vi "_sp_spurious.vi"(11 "SP_Spurious":cluster{"Rx_output_data":path, "SAVE":bool}={"Rx_output_data"=path "L:/cartridge/assembly/SN03/03-23/111227_DSB/SP_810.00_120_111227_CCA03-23_DSBFB.csv", "SAVE"=TRUE}) -> (1 "出力文字列":string="SP_spurious,0.82,4.01,-33.89,-32.15 ")   [LabVIEW 2017]
uses:
  <vilib>/Utility/file.llb/Read From Spreadsheet File (string).vi
panel:
  out "配列 2":dbl[][](array[numeric])=[[3.8, -17.12272, -18.81083, -15.55195, -27.42913, -0.8529618823529413, 2646.4699989426, 27.159200000349998, 21.830696906606043], [3.85, -17.57263, -19.57423, -15.61331, -27.39271, -0.8547822352941177, 2630.0700003280003, 27.222799998728, 21.827656711269793], [3.9, -17.18393, -19.46044, -15.25915, -26.95194, -0.8662073529411765, 2669.6499992084, 27.104500002366002, 21.82485128829734], [3.95, -16.20817, -18.50417, -14.57025, -26.2268, -0.8667218823529415, 2730.9599987738, 27.08000000049, 21.822294447827726], [4.0, -15.03429, -17.26599, -13.90883, -25.64848, -0.882467, 2669.1500012362003, 27.084199999916, 21.82], [4.05, -14.82404, -17.0148, -13.89065, -25.63071, -0.881857, 2537.9100026248, 27.120499999274, 21.817975444814163], [4.1, -14.67198, -16.88321, -13.75199, -25.74328, -0.8925589411764706, 2521.6700003248, 26.984300002724, 21.81620304171403], [4.15, -13.82526, -16.05723, -13.35155, -25.22083, -0.8985360624999998, 2529.2999998474, 26.948000000726, 21.81465874000436], [4.2, -13.29308, -15.43659, -13.22012, -25.15282, -0.901060705882353, 2508.1700004226, 26.933300000294, 21.81331848898993], [4.25, -13.22027, -15.33436, -13.24037, -25.05297, -0.9175218823529412, 2527.4499996144, 26.893400000798, 21.812158237975495], [4.3, -13.31871, -15.44813, -13.02047, -24.85233, -0.9171115294117648, 2617.4499981999998, 26.800200001864, 21.81115393626583], [4.35, -13.69981, -15.96198, -12.64103, -24.38364, -0.9331128235294116, 2655.3199992426003, 26.946899997065998, 21.810281533165693], [4.4, -13.88617, -16.39624, -12.56773, -24.29817, -0.9225989999999998, 2612.6100008542003, 26.89840000097, 21.809516977979857], [4.45, -14.02675, -16.71935, -12.80309, -24.58885, -0.9326420000000001, 2578.7800006766, 26.85540000086, 21.808836220013085], [4.5, -14.20917, -16.89711, -12.97901, -24.88372, -0.9390088823529412, 2494.6900016818004, 26.752700002054002, 21.808215208570147], [4.55, -14.08214, -16.69081, -12.94844, -24.93315, -0.948472375, 2435.9600011746, 26.64920000207, 21.807629892955802], [4.6, -14.17748, -16.75517, -13.06879, -25.00575, -0.9494775294117647, 2433.2400000544, 26.427400004436, 21.80705622247482], [4.65, -14.20809, -16.81901, -13.13087, -25.16717, -0.9524575882352941, 2443.0399998039998, 26.363500001278, 21.80647014643197], [4.7, -13.73884, -16.38887, -13.13099, -25.03512, -0.9655740588235294, 2433.8500001838, 26.45199999823, 21.805847614132016], [4.75, -13.52419, -16.15298, -13.15192, -24.9704, -0.9653059411764703, 2516.0199983566, 26.454299999954, 21.805164574879722], [4.8, -13.5663, -16.20232, -13.10517, -24.80095, -0.976770176470588, 2562.8099990642, 26.343600002214, 21.804396977979856], [4.85, -13.97629, -16.65383, -13.30715, -25.25404, -0.9746549411764707, 2478.4000016882, 26.311400000644, 21.803520772737187], [4.9, -14.61364, -17.38417, -13.78671, -25.66877, -0.988881117647059, 2394.9800016684003, 26.140100003426, 21.802511908456477], [4.95, -14.4268, -17.25931, -13.81209, -25.80221, -0.9904888125, 2426.7199993652, 26.145399999894, 21.801346334442492], [5.0, -13.84685, -16.67325, -13.20797, -25.09457, -0.9986477647058825, 2402.3700004869997, 26.405599994796, 21.8], [5.05, -14.28601, -17.05717, -13.45101, -25.54052, -1.004, 2304.7500019524, 26.325300001606, 21.798457844989954], [5.1, -14.91876, -17.64101, -13.96415, -26.02207, -1.0068823529411761, 2324.9199995966, 26.481899996868, 21.796740771498058], [5.15, -15.14906, -17.85047, -14.16308, -26.17572, -1.0180588235294117, 2408.1599983352, 26.271100004216002, 21.794878672166195], [5.2, -14.66069, -17.39484, -13.82115, -25.80543, -1.0208823529411764, 2393.2200002987997, 26.329699998827998, 21.792901439636257], [5.25, -13.73691, -16.45963, -13.31747, -25.36704, -1.028, 2326.370001337, 26.25120000157, 21.790838966550133], [5.3, -13.70664, -16.41934, -13.34713, -25.41262, -1.0291176470588232, 2366.9299991887997, 26.28519999932, 21.78872114554971], [5.35, -14.26567, -16.97919, -13.7311, -25.69348, -1.042, 2383.6799996649997, 26.357999998544, 21.78657786927688], [5.4, -14.42577, -17.17993, -13.89956, -26.00954, -1.046, 2311.580001442, 26.332800000503997, 21.784439030373523], [5.45, -14.3035, -17.10186, -13.87839, -26.01249, -1.0538235294117648, 2274.08000075, 26.241800001820003, 21.782334521481534], [5.5, -14.13436, -16.92141, -13.94402, -26.09274, -1.0542500000000001, 2305.5199993712, 26.224000000356, 21.780294235242803], [5.55, -14.09064, -16.88934, -13.93655, -25.97309, -1.0640588235294117, 2314.2099998262, 26.143600001608, 21.778348064299216], [5.6, -14.13487, -16.88146, -13.83602, -26.02727, -1.0725882352941176, 2258.5000011142, 26.194499998982, 21.776525901292658], [5.65, -14.0179, -16.75543, -13.67357, -25.85477, -1.0641764705882353, 2249.6300001774002, 26.303699997816, 21.774857638865026], [5.7, -13.742, -16.4761, -13.49645, -25.65245, -1.085294117647059, 2312.4099987443997, 26.495899996156, 21.7733731696582], [5.75, -13.63401, -16.37811, -13.62051, -25.66763, -1.0879411764705882, 2296.9000003102, 26.546799998982, 21.77210238631407], [5.8, -13.9966, -16.7347, -14.08119, -26.28417, -1.0975294117647059, 2229.90000134, 26.494200001052, 21.77107518147453], [5.85, -14.3776, -17.12208, -14.29554, -26.5205, -1.0957647058823532, 2219.9900001981996, 26.459700000690002, 21.770321447781463], [5.9, -14.33998, -17.0836, -14.21864, -26.41191, -1.0961250000000002, 2230.8999997818, 26.353800002118, 21.76987107787676], [5.95, -14.05573, -16.80771, -13.83659, -26.01129, -1.106764705882353, 2262.3899993702, 26.544199996192, 21.76975396440231], [6.0, -14.15222, -16.88773, -14.02318, -26.27665, -1.110529411764706, 2218.8600008706003, 26.523000000424, 21.77], [6.05, -14.42877, -17.16834, -14.46916, -26.71696, -1.1207647058823527, 2201.7700003418, 26.482100000818, 21.770629425226016], [6.1, -14.82458, -17.54857, -14.74361, -26.94142, -1.1145882352941179, 2213.8099997592, 26.528199999077998, 21.77162387229374], [6.15, -14.43141, -17.15023, -14.50576, -26.74506, -1.1284117647058822, 2219.209999892, 26.454400001476, 21.77295532133086], [6.2, -13.88065, -16.61938, -14.37111, -26.68039, -1.128235294117647, 2179.0500008032004, 26.372000001648, 21.77459575246504], [6.25, -13.64365, -16.3979, -14.22502, -26.5427, -1.135764705882353, 2168.7100002068, 26.34000000064, 21.77651714582397], [6.3, -13.8741, -16.64741, -14.49609, -26.71762, -1.14025, 2200.3899993664, 26.582799995143997, 21.77869148153533], [6.35, -14.26957, -17.0322, -14.86186, -27.19956, -1.1440588235294114, 2204.6199999154, 26.591799999819997, 21.781090739726796], [6.4, -15.05829, -17.80809, -15.42064, -27.71206, -1.1539411764705882, 2184.0000004124, 26.470100002434, 21.78368690052605], [6.45, -14.96881, -17.71266, -15.38201, -27.65482, -1.1564705882352941, 2195.249999775, 26.481999999762, 21.786451944060772], [6.5, -14.62204, -17.38934, -15.02896, -27.20097, -1.1578823529411766, 2242.3699990575997, 26.306800003503998, 21.789357850458643], [6.55, -14.93231, -17.69407, -15.10335, -27.40647, -1.164235294117647, 2205.1300007448003, 26.310299999930002, 21.79237659984734], [6.6, -15.6833, -18.43714, -15.87043, -28.20904, -1.172, 2152.5300010520004, 26.339899999408, 21.795480172354544], [6.65, -16.11679, -18.87216, -16.20987, -28.58401, -1.1799411764705883, 2167.9899996908, 26.356799999661998, 21.798640548107933], [6.7, -15.71971, -18.45462, -15.76916, -28.0619, -1.185, 2201.939999321, 26.396499999206, 21.80182970723519], [6.75, -15.0464, -17.78941, -15.52487, -27.82688, -1.195, 2182.7000003847998, 26.399599999938, 21.805019629863992], [6.8, -15.48116, -18.24106, -16.05464, -28.38039, -1.2004117647058823, 2165.3400003472, 26.28360000232, 21.808182296122023], [6.85, -16.22272, -18.99162, -16.63654, -28.97924, -1.201, 2225.439998798, 26.274900000174, 21.81128968613696], [6.9, -15.67766, -18.42345, -16.38983, -28.69264, -1.2098823529411764, 2234.0299998282003, 26.270200000094, 21.814313780036482], [6.95, -15.36656, -18.07411, -15.9862, -28.27599, -1.2114117647058824, 2165.6200013682, 26.381899997766002, 21.817226557948267], [7.0, -15.74528, -18.46492, -16.29495, -28.63586, -1.218, 2163.1900000486003, 26.272700002184, 21.82], [7.05, -16.00173, -18.75385, -16.78861, -29.11719, -1.2230588235294118, 2187.8999995058, 26.169500002063998, 21.82260695410598], [7.1, -15.95475, -18.70909, -16.46813, -28.80718, -1.2295882352941179, 2186.0500000370002, 26.233599998718, 21.825023739326973], [7.15, -15.74736, -18.51188, -16.0888, -28.41011, -1.228, 2172.6600002677997, 26.140200001868, 21.827227542510375], [7.2, -15.79896, -18.55205, -16.49574, -28.80938, -1.2389411764705882, 2190.1299996506, 26.035800002088, 21.82919555050358], [7.25, -16.55221, -19.29029, -17.09613, -29.38037, -1.2441250000000001, 2230.579999191, 25.944300001829998, 21.830904950153982], [7.3, -16.63515, -19.36656, -17.1755, -29.45088, -1.2501764705882352, 2201.3800005840003, 26.127399996338003, 21.83233292830897], [7.35, -16.28817, -19.02285, -17.12399, -29.45578, -1.2507058823529413, 2186.5600002964, 26.014300002261997, 21.833456671815934], [7.4, -15.91257, -18.66145, -16.74209, -29.02037, -1.2591176470588235, 2205.0399996304, 26.029399999698, 21.834253367522273], [7.45, -15.41844, -18.14403, -16.48895, -28.79334, -1.2650588235294118, 2206.9099999626, 25.964200001304, 21.83470020227537], [7.5, -15.41264, -18.10839, -16.57757, -28.91563, -1.273764705882353, 2195.2200002338, 26.019099998902, 21.834774362922627], [7.55, -15.98175, -18.66501, -16.9447, -29.22746, -1.2748235294117647, 2200.019999904, 25.824000003902, 21.834453036311427], [7.6, -15.94066, -18.66749, -17.16323, -29.42903, -1.2809411764705882, 2244.7899991045997, 25.813600000208, 21.833713409289167], [7.65, -15.86338, -18.63036, -17.30867, -29.55716, -1.2772500000000002, 2247.2699999504, 25.856499999142, 21.83253266870324], [7.7, -15.93995, -18.73317, -17.33017, -29.58961, -1.2859411764705884, 2238.1100001832, 25.730900002511998, 21.83088800140104], [7.75, -15.60121, -18.40257, -17.32444, -29.63481, -1.299588235294118, 2218.8700003848, 25.69040000081, 21.828756594229954], [7.8, -15.52939, -18.3085, -17.34604, -29.61109, -1.2968235294117643, 2243.669999504, 25.680500000198, 21.82611563403738], [7.85, -15.91931, -18.69063, -17.7087, -29.96924, -1.3002352941176467, 2245.9399999546, 25.647100000667997, 21.8229423076707], [7.9, -16.06734, -18.84154, -18.21152, -30.51118, -1.3056250000000003, 2218.990000539, 25.507500002792, 21.819213801977316], [7.95, -16.2394, -19.01631, -18.39538, -30.77489, -1.313764705882353, 2222.539999929, 25.53849999938, 21.81490730380462], [8.0, -16.0832, -18.82693, -18.18621, -30.42877, -1.3231176470588235, 2253.7699993754, 25.421100002348, 21.81], [8.05, -15.9397, -18.65948, -18.21682, -30.46989, -1.332941176470588, 2276.81, 25.2307, 21.804486508350074], [8.1, -16.44804, -19.16853, -18.58308, -30.82861, -1.335, 2261.15, 25.2839, 21.79843117039837], [8.15, -16.97081, -19.72537, -19.0693, -31.4089, -1.3383529411764703, 2262.78, 25.2973, 21.79191575862764], [8.2, -16.87192, -19.67071, -19.41342, -31.67662, -1.348647058823529, 2301.63, 25.0593, 21.78502204552063], [8.25, -17.21139, -20.03537, -19.67853, -31.95149, -1.3514117647058825, 2289.19, 24.9943, 21.777831803560098], [8.3, -17.29203, -20.11014, -19.70503, -32.02495, -1.352470588235294, 2259.82, 25.224, 21.77042680522879], [8.35, -16.73358, -19.52565, -19.51154, -31.79005, -1.357705882352941, 2266.94, 24.9458, 21.76288882300946], [8.4, -16.47973, -19.26356, -19.55496, -31.8567, -1.365235294117647, 2296.06, 24.8175, 21.75529962938486], [8.45, -16.96765, -19.74245, -20.13428, -32.43519, -1.3692499999999999, 2317.78, 24.8136, 21.747740996837745], [8.5, -17.89289, -20.67773, -21.16278, -33.47596, -1.377, 2296.65, 24.8236, 21.740294697850857], [8.55, -18.31942, -21.11132, -21.53435, -33.99178, -1.377882352941177, 2303.42, 24.7167, 21.73304250490695], [8.6, -17.91342, -20.68657, -21.06001, -33.3284, -1.3864117647058825, 2312.28, 24.5475, 21.72606619048878], [8.65, -17.50286, -20.31712, -20.86753, -33.1991, -1.3915882352941176, 2326.39, 24.57, 21.719447527079094], [8.7, -17.7744, -20.60603, -21.46811, -33.89479, -1.3978823529411766, 2298.81, 24.1647, 21.713268287160645], [8.75, -17.86462, -20.69869, -21.66053, -34.15056, -1.4036470588235284, 2302.5, 24.3807, 21.707610243216184], [8.8, -17.71743, -20.57318, -21.35601, -33.74465, -1.4073529411764707, 2313.14, 24.5441, 21.702555167728462], [8.85, -17.94226, -20.78062, -21.59592, -34.02443, -1.4161875, 2345.93, 24.4626, 21.698184833180232], [8.9, -18.34472, -21.16955, -22.16719, -34.56456, -1.4160588235294116, 2339.53, 24.3008, 21.694581012054247], [8.95, -18.04812, -20.86419, -21.99622, -34.46492, -1.4309411764705886, 2338.73, 24.441, 21.69182547683325], [9.0, -17.40652, -20.21983, -21.48231, -33.78672, -1.4215882352941176, 2358.4, 24.3139, 21.69], [9.05, -17.24231, -20.07737, -21.48494, -33.82899, -1.4349411764705877, 2366.74, 24.1072, 21.689155762493723], [9.1, -17.74864, -20.56868, -21.94918, -34.39316, -1.4335882352941178, 2338.76, 24.3848, 21.689221579079543], [9.15, -18.4194, -21.25906, -22.30343, -34.74111, -1.453, 2315.94, 24.6737, 21.690095672979066], [9.2, -18.22584, -21.06735, -22.19776, -34.35875, -1.451705882352941, 2343.85, 24.5305, 21.69167626741389], [9.25, -17.60283, -20.47247, -21.72121, -33.8754, -1.4561250000000001, 2374.94, 24.293, 21.69386158560562], [9.3, -17.285, -20.1526, -21.26908, -33.42764, -1.4694117647058822, 2365.34, 24.4681, 21.69654985077586], [9.35, -17.46603, -20.32564, -21.38399, -33.71154, -1.4681764705882352, 2354.91, 24.3401, 21.699639286146212], [9.4, -17.69275, -20.52774, -21.7712, -34.03559, -1.4925882352941173, 2368.34, 24.4059, 21.703028114938277], [9.45, -17.89483, -20.70066, -21.80327, -33.93689, -1.473, 2362.78, 24.6405, 21.706614560373655], [9.5, -17.75022, -20.53087, -21.69907, -34.00557, -1.507411764705883, 2338.42, 24.6167, 21.710296845673955], [9.55, -17.66432, -20.45212, -21.90227, -34.10663, -1.4951764705882342, 2333.22, 24.5527, 21.713973194060774], [9.6, -17.65736, -20.44671, -21.78109, -33.9852, -1.522470588235294, 2332.23, 24.4424, 21.717541828755717], [9.65, -17.73314, -20.5128, -21.7289, -33.99685, -1.517823529411764, 2328.62, 24.6084, 21.720900972980388], [9.7, -17.4669, -20.25952, -21.67133, -33.91276, -1.525588235294116, 2351.26, 24.2804, 21.723948849956383], [9.75, -17.76851, -20.58019, -22.0069, -34.18419, -1.5647058823529412, 2359.86, 24.4864, 21.72658368290531], [9.8, -18.45745, -21.3164, -22.66344, -34.81685, -1.5282499999999999, 2394.51, 24.4116, 21.72870369504877], [9.85, -18.74849, -21.60512, -23.1135, -35.51059, -1.5908235294117645, 2378.32, 24.3508, 21.73020710960837], [9.9, -18.03912, -20.85912, -22.19721, -34.52363, -1.5453529411764708, 2394.59, 24.2431, 21.730992149805704], [9.95, -17.9064, -20.68631, -21.64287, -33.76706, -1.6109999999999993, 2382.76, 24.4119, 21.730957038862382], [10.0, -18.76585, -21.52492, -22.34931, -34.56586, -1.5900588235294104, 2349.48, 24.4835, 21.73], [10.05, -19.5962, -22.32853, -22.9941, -35.31366, -1.6072352941176506, 2367.23, 24.3783, 21.72805419167504], [10.1, -19.6706, -22.4559, -22.82671, -35.05968, -1.6390588235294121, 2371.78, 24.5145, 21.72519251328346], [10.15, -19.60253, -22.38713, -22.75759, -35.06578, -1.594882352941177, 2400.96, 24.3435, 21.721522799456107], [10.2, -19.78752, -22.57098, -23.06087, -35.44369, -1.681875, 2420.45, 24.0411, 21.71715288482381], [10.25, -20.0526, -22.84692, -23.63574, -35.82155, -1.6011764705882354, 2439.32, 23.8385, 21.712190604017422], [10.3, -19.54974, -22.37162, -23.29077, -35.54749, -1.6889411764705888, 2425.46, 24.0043, 21.70674379166777], [10.35, -19.60772, -22.45374, -23.18082, -35.44497, -1.6339411764705871, 2402.21, 24.136, 21.700920282405693], [10.4, -19.77289, -22.58667, -23.44011, -35.6872, -1.6639411764705916, 2403.53, 24.1481, 21.69482791086204], [10.45, -19.79049, -22.58858, -23.37076, -35.6931, -1.6936470588235286, 2410.86, 24.2845, 21.688574511667635], [10.5, -19.04526, -21.81113, -22.73856, -34.75031, -1.6280000000000006, 2432.24, 24.1535, 21.68226791945333], [10.55, -18.56993, -21.3308, -22.71269, -34.42597, -1.7282941176470574, 2457.87, 23.9651, 21.676015968849956], [10.6, -18.81393, -21.59022, -23.3418, -35.09374, -1.627000000000001, 2472.89, 23.7868, 21.669926494488355], [10.65, -19.22983, -22.00177, -23.51241, -35.50699, -1.7109411764705882, 2463.24, 23.8037, 21.664107330999364], [10.7, -19.31875, -22.05797, -23.32962, -35.59218, -1.6540588235294145, 2430.32, 23.8234, 21.658666313013825], [10.75, -19.05511, -21.80451, -23.11849, -35.37068, -1.6625882352941161, 2456.31, 23.8229, 21.653711275162575], [10.8, -19.3566, -22.10467, -23.36395, -35.42174, -1.644, 2526.85, 23.8448, 21.64935005207645], [10.85, -19.0206, -21.80983, -23.26736, -35.08837, -1.653941176470586, 2539.44, 23.6902, 21.645690478386292], [10.9, -18.31242, -21.08287, -22.35121, -34.319, -1.678058823529411, 2516.98, 23.7731, 21.642840388722938], [10.95, -18.58308, -21.32811, -22.20398, -34.26554, -1.6376470588235292, 2511.94, 23.7372, 21.64090761771723], [11.0, -19.33065, -22.06466, -22.81771, -34.93946, -1.6834705882352938, 2495.74, 23.8567, 21.64], [11.05, -19.70611, -22.43568, -23.07443, -35.23765, -1.6487058823529408, 2471.76, 23.7069, 21.64017747080613], [11.1, -19.03199, -21.75445, -22.37182, -34.36297, -1.6840588235294118, 2484.68, 23.978, 21.64130836778662], [11.15, -18.20851, -20.94228, -21.81273, -33.92755, -1.65975, 2530.13, 23.6561, 21.643213129196518], [11.2, -18.60047, -21.36138, -22.13935, -34.33841, -1.7035294117647042, 2549.97, 23.6568, 21.645712193290862], [11.25, -19.51813, -22.27067, -22.85502, -34.9773, -1.6814705882352947, 2588.62, 23.5463, 21.6486259983247], [11.3, -20.00388, -22.73884, -23.1136, -35.31568, -1.7118823529411817, 2547.84, 23.759, 21.651774982553068], [11.35, -20.09303, -22.81332, -23.00719, -35.05995, -1.7251176470588228, 2534.41, 23.8176, 21.654979584231015], [11.4, -19.73824, -22.45692, -22.58862, -34.67323, -1.7182352941176506, 2543.99, 23.8915, 21.658060241613576], [11.45, -19.50205, -22.22064, -22.28212, -34.3972, -1.75829411764706, 2558.35, 23.9421, 21.660837392955802], [11.5, -19.44096, -22.15222, -22.1292, -34.22024, -1.7096470588235253, 2566.32, 23.8669, 21.663131476512728], [11.55, -19.53986, -22.21978, -22.16747, -34.08258, -1.805937499999999, 2585.21, 23.691, 21.664762930539403], [11.6, -19.66825, -22.31744, -22.50284, -34.28826, -1.7306470588235299, 2620.79, 23.6435, 21.665552193290864], [11.65, -20.25282, -22.89179, -22.68607, -34.6127, -1.833705882352942, 2632.79, 23.8005, 21.665319703022153], [11.7, -20.71909, -23.33487, -22.77796, -34.75574, -1.7838235294117686, 2608.38, 23.9055, 21.663885897988315], [11.75, -20.60419, -23.22526, -22.42747, -34.3851, -1.7971764705882394, 2594.61, 24.0102, 21.661071216444395], [11.8, -19.96298, -22.55664, -21.58718, -33.45363, -1.8430588235294112, 2639.94, 23.9067, 21.656696096645433], [11.85, -19.76787, -22.40006, -21.42269, -33.29006, -1.7760588235294126, 2643.51, 23.9414, 21.650580976846467], [11.9, -20.8505, -23.49592, -22.22725, -34.22635, -1.8767647058823524, 2626.67, 23.9677, 21.642546295302548], [11.95, -21.60192, -24.17152, -22.54207, -34.5773, -1.7737499999999975, 2639.97, 23.9508, 21.63241249026871], [12.0, -21.64507, -24.22899, -22.299, -34.30385, -1.8910588235294117, 2735.39, 23.7742, 21.62], [12.05, -21.23121, -23.79945, -21.79121, -33.84, -1.7987058823529407, 2735.72, 24.015, 21.60517967510045], [12.1, -20.95311, -23.50938, -21.58213, -33.39882, -1.879823529411763, 2675.38, 24.0166, 21.588024015570067], [12.15, -20.98547, -23.59292, -21.93953, -33.86782, -1.885, 2668.38, 24.2213, 21.56865593375783], [12.2, -20.95372, -23.58369, -22.31312, -34.16981, -1.8179411764705862, 2763.59, 23.8837, 21.54719834201274]]
  in  "タブ制御器":enum32{"YIGファイル", "配列"}(tab)
  out "Totalband Power":dbl=-32.14616354917376 format="%#_4g"
  out "Inband Power":dbl=-33.891453586938624 format="%#_4g"
  out "max":dbl=0.820999999999998 format="%#_5g"
  out "XYグラフ 7":cluster{"データ配列":dbl[], "データ配列":dbl[]}[](graph)
  out "Inband PP":dbl=4.009999999999991 format="%#_4g"
  out "配列":dbl[][](array[numeric])
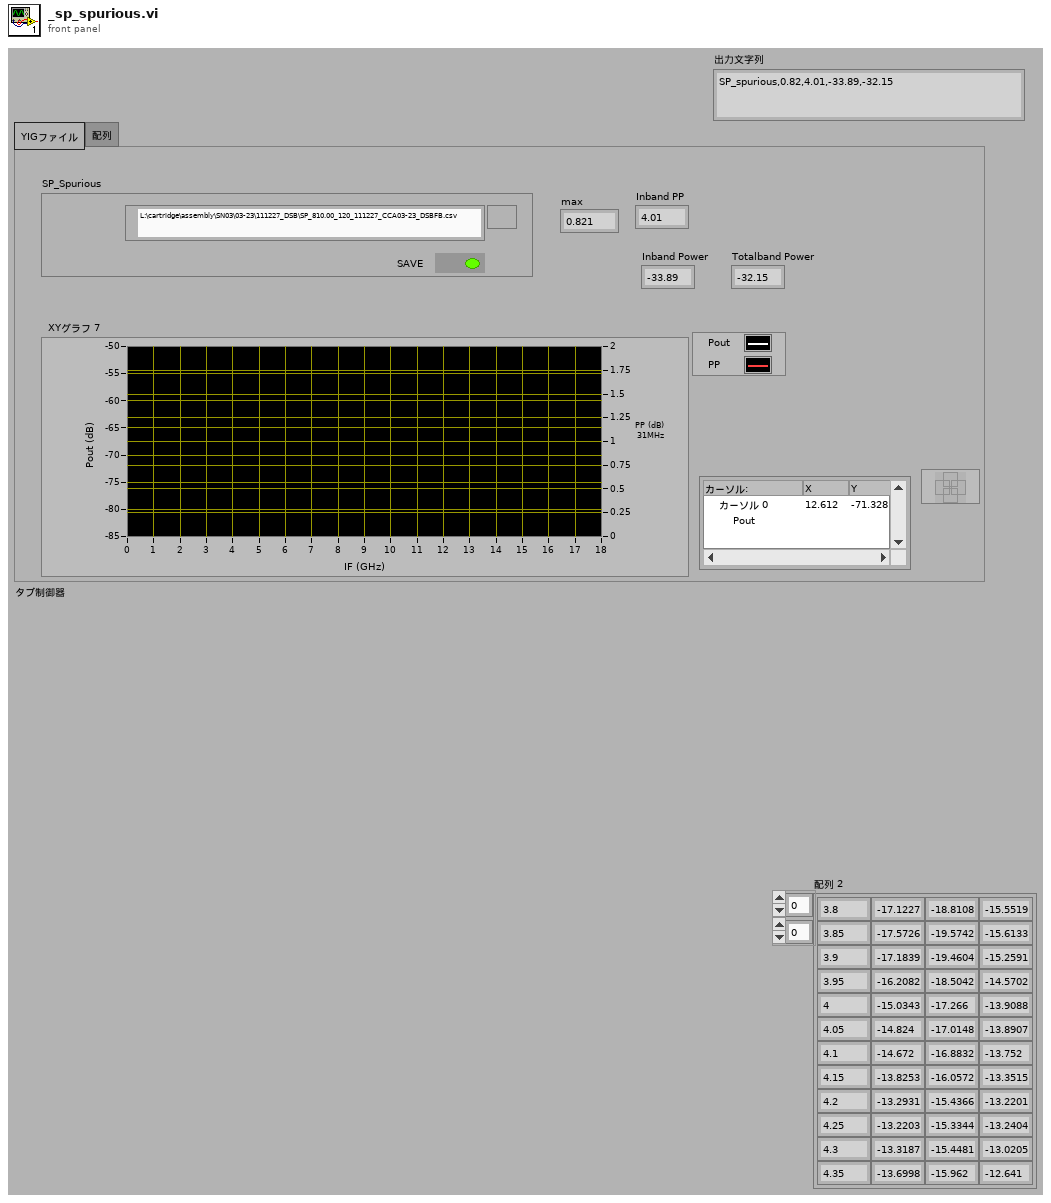
[diagram p1: front panel]
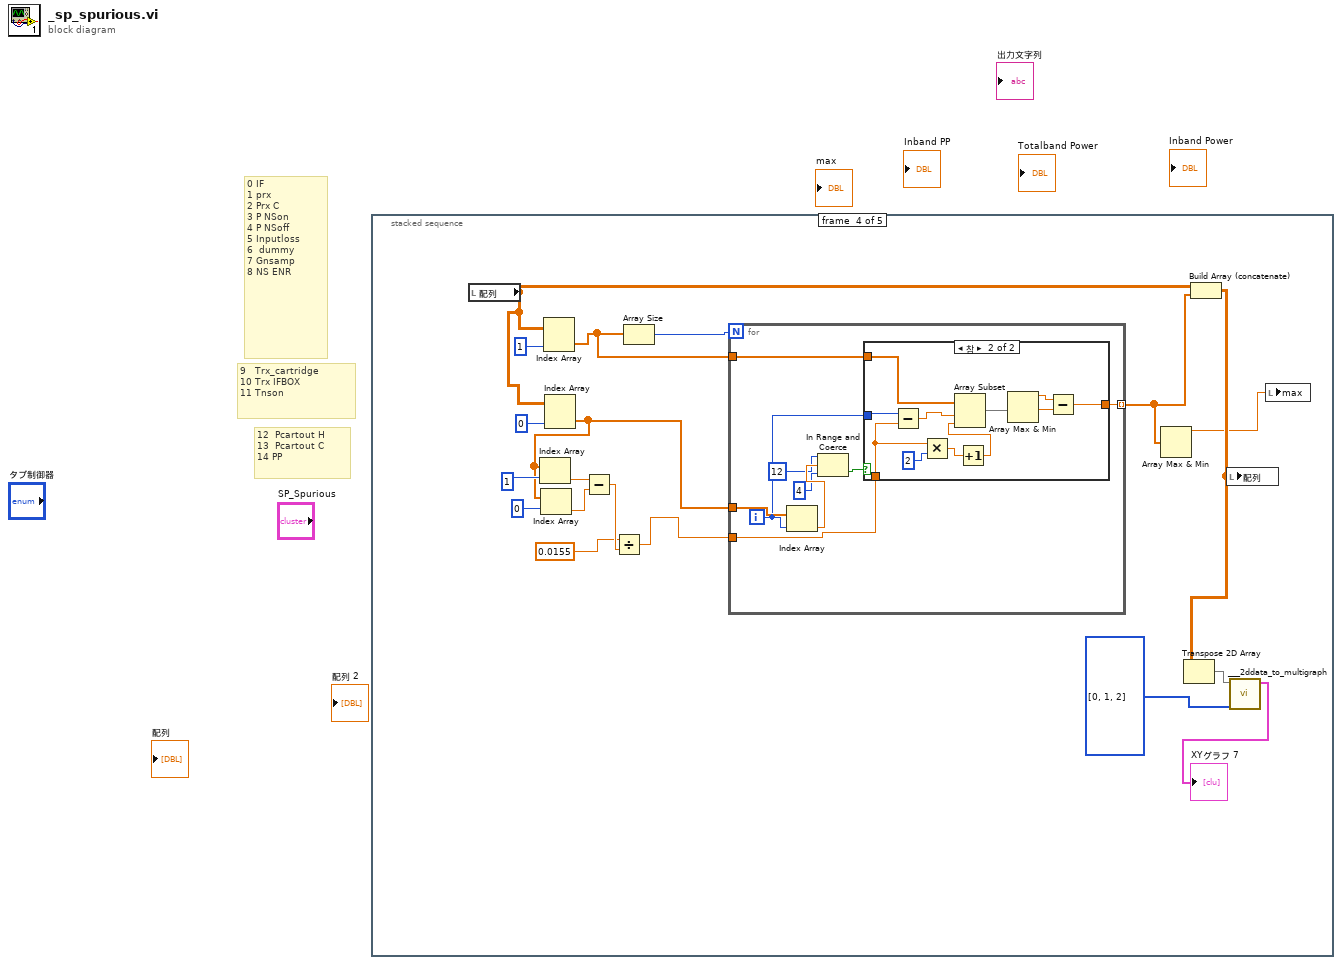
[diagram p0: block diagram]
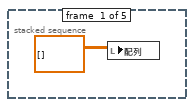
[diagram p2: hidden frame]
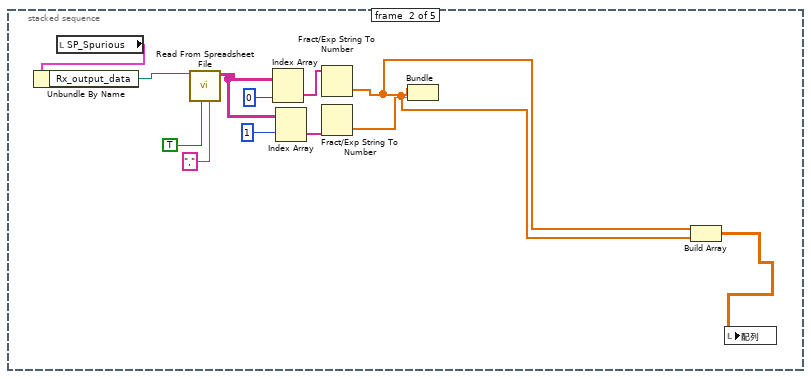
[diagram p3: hidden frame]
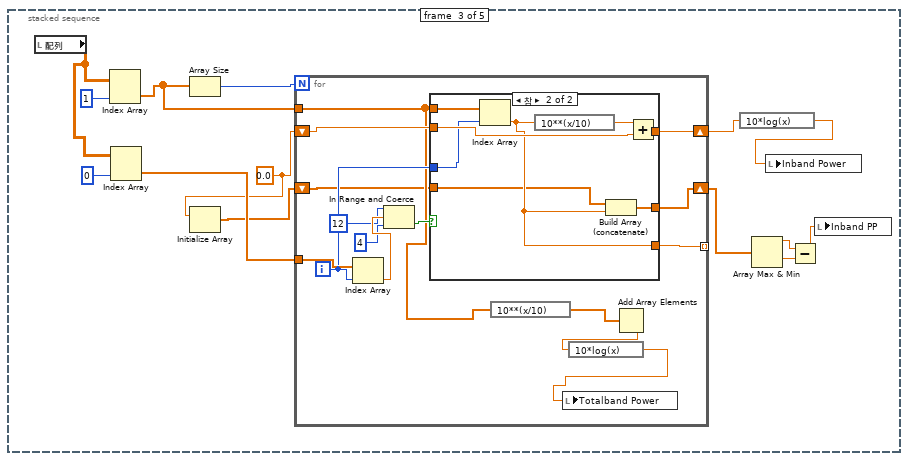
[diagram p4: hidden frame]
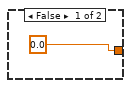
[diagram p6: hidden frame]
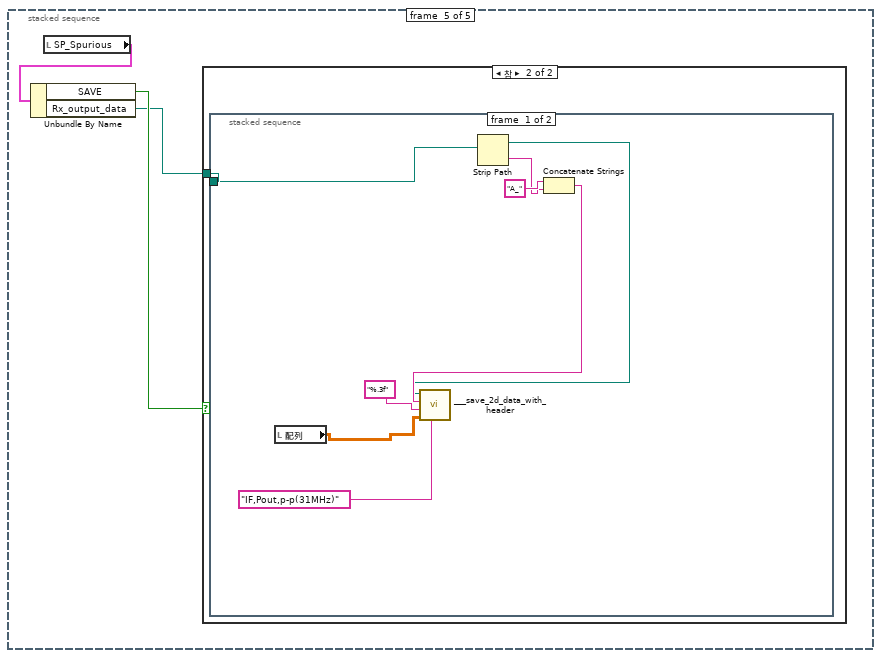
[diagram p7: hidden frame]
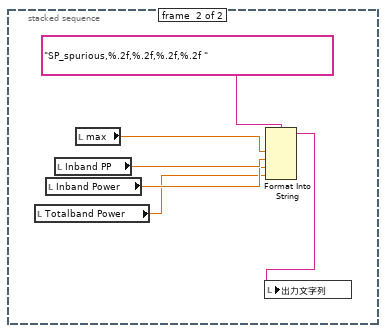
[diagram p9: hidden frame]
diagram:
  # "12  Pcartout H\n13  Pcartout C\n14 PP"
  # "9   Trx_cartridge\n10 Trx IFBOX\n11 Tnson"
  # "0 IF\n1 prx\n2 Prx C\n3 P NSon\n4 P NSoff\n5 Inputloss\n6  dummy\n7 Gnsamp\n8 NS ENR"
  n1 = stacked-sequence {
    frame #0 {
      n2 = local write "配列"(dbl[][] []) -> ()
    }
    frame #1 {
      n3 = local read "SP_Spurious"() -> (w2:cluster{"Rx_output_data":path, "SAVE":bool})
      n4 = Unbundle By Name(w2) -> ("Rx_output_data"=w8:path)
      n5 = call-poly <vilib>:"Read From Spreadsheet File.vi"("delimiter (\\t)"=",", "transpose (no:F)"=TRUE, "file path (dialog if empty)"=w8) -> ("all rows"=w3:string[][])  [unwired: 4 in, 4 out]
      n6 = Index Array(array=w3, index (row)=0) -> (element=w7:string[])  [unwired: 1 in]
      n7 = Index Array(array=w3, index (row)=1) -> (element=w5:string[])  [unwired: 1 in]
      n8 = Fract/Exp String To Number(string=w7) -> (number=w6:dbl[])  [unwired: 3 in, 1 out]
      n9 = Fract/Exp String To Number(string=w5) -> (number=w4:dbl[])  [unwired: 3 in, 1 out]
      n10 = Bundle(w6, w4) -> ()  [unwired: 1 in, 1 out]
      n11 = Build Array(w6, w4) -> (w9:dbl[][])
      n12 = local write "配列"(w9) -> ()
    }
    frame #2 {
      w16 = 0.0
      n13 = local read "配列"() -> (w22:dbl[][])
      n14 = Index Array(array=w22, index (row)=1) -> (element=w23:dbl[])  [unwired: 1 in]
      n15 = Index Array(array=w22, index (row)=0) -> (element=w24:dbl[])  [unwired: 1 in]
      n16 = Array Size(array=w23) -> (size(s)=w26:i32)
      n17 = Initialize Array(w16) -> (w15:dbl[])  [unwired: 1 in]
      n18 = for {
        N: w26 -> [_]
        tunnel: w24 -> [w42]
        shift-right: [w35] -> w18
        shift-left: w16 -> [w36]
        tunnel: w23 -> [w33]
        tunnel: [w34] -> _ mode=indexing
        shift-right: [w29] -> w14
        shift-left: w15 -> [w28]
        i -> [w37]
        n19 = Index Array(array=w42, index=w37) -> (element=w41:dbl)
        n20 = In Range and Coerce(upper limit=12, x=w41, lower limit=4) -> (In Range?=w38:bool)  [unwired: 1 out]
        n21 = case shown="참" w38 {
          tunnel: w37 -> [_ w48]
          tunnel: w36 -> [w44 w49]
          tunnel: [w44 w50] -> w35
          tunnel: w33 -> [_ w51]
          tunnel: [_ w47] -> w34
          tunnel: [w43 w46] -> w29
          tunnel: w28 -> [w43 w45]
          frame False {
          }
          frame True {
            n22 = Index Array(array=w51, index=w48) -> (element=w47:dbl)
            n23 = expression code="10**(x/10)"(w47) -> (w52:dbl)
            n24 = Build Array (concatenate)(w45, w47) -> (w46:dbl[])
            n25 = Add(x=w52, y=w49) -> (x+y=w50:dbl)
          }
        }
        n26 = expression code="10**(x/10)"(w33) -> (w32:dbl[])
        n27 = Add Array Elements(numeric array=w32) -> (sum=w31:dbl)
        n28 = expression code="10*log(x)"(w31) -> (w30:dbl)
        n29 = local write "Totalband Power"(w30) -> ()
      }
      n30 = expression code="10*log(x)"(w18) -> (w17:dbl)
      n31 = Array Max & Min(array=w14) -> (max value=w21:dbl, min value=w20:dbl)  [unwired: 2 out]
      n32 = local write "Inband Power"(w17) -> ()
      n33 = Subtract(x=w21, y=w20) -> (x-y=w19:dbl)
      n34 = local write "Inband PP"(w19) -> ()
    }
    frame #3 {
      n35 = local read "配列"() -> (w62:dbl[][])
      n36 = Index Array(array=w62, index (row)=1) -> (element=w63:dbl[])  [unwired: 1 in]
      n37 = Index Array(array=w62, index (row)=0) -> (element=w66:dbl[])  [unwired: 1 in]
      n38 = Index Array(array=w66, index=1) -> (element=w65:dbl)
      n39 = Index Array(array=w66, index=0) -> (element=w64:dbl)
      n40 = Subtract(x=w65, y=w64) -> (x-y=w54:dbl)
      n41 = Divide(x=0.0155, y=w54) -> (x/y=w55:dbl)
      n42 = Array Size(array=w63) -> (size(s)=w70:i32)
      n43 = for {
        N: w70 -> [_]
        tunnel: w66 -> [w80]
        tunnel: w63 -> [w74]
        tunnel: w55 -> [w73]
        tunnel: [w72] -> w57 mode=indexing
        i -> [w75]
        n44 = Index Array(array=w80, index=w75) -> (element=w79:dbl)
        n45 = In Range and Coerce(upper limit=12, x=w79, lower limit=4) -> (In Range?=w76:bool)  [unwired: 1 out]
        n46 = case shown="참" w76 {
          tunnel: w75 -> [_ w91]
          tunnel: w74 -> [_ w92]
          tunnel: w73 -> [_ w89]
          tunnel: [0.0 w85] -> w72
          frame False {
          }
          frame True {
            n47 = Subtract(x=w91, y=w89) -> (x-y=w90:dbl)
            n48 = Multiply(x=w89, y=2) -> (x*y=w84:dbl)
            n49 = Increment(x=w84) -> (x+1=w83:dbl)
            n50 = Array Subset(array=w92, index=w90, length=w83) -> (w88:dbl[])
            n51 = Array Max & Min(array=w88) -> (max value=w87:dbl, min value=w86:dbl)  [unwired: 2 out]
            n52 = Subtract(x=w87, y=w86) -> (x-y=w85:dbl)
          }
        }
      }
      n53 = Array Max & Min(array=w57) -> (max value=w56:dbl)  [unwired: 3 out]
      n54 = Build Array (concatenate)(w62, w57) -> (w58:dbl[][])
      n55 = Transpose 2D Array(2D array=w58) -> (transposed array=w59:dbl[][])
      n56 = local write "配列"(w58) -> ()
      n57 = call "___2ddata_to_multigraph.vi"("列"=i32[] [0, 1, 2], "データ配列"=w59) -> ("XYグラフ"=→"XYグラフ 7":cluster{"データ配列":dbl[], "データ配列":dbl[]}[])  [unwired: 5 in]
      n58 = local write "max"(w56) -> ()
    }
    frame #4 {
      n59 = local read "SP_Spurious"() -> (w93:cluster{"Rx_output_data":path, "SAVE":bool})
      n60 = Unbundle By Name(w93) -> ("SAVE"=w95:bool, "Rx_output_data"=w94:path)
      n61 = case shown="참" w95 {
        tunnel: w94 -> [_ w96]
        frame False {
        }
        frame True {
          n62 = stacked-sequence {
            tunnel: w96 -> [w97 _]
            frame #0 {
              n63 = local read "配列"() -> (w102:dbl[][])
              n64 = Strip Path(path=w97) -> (stripped path=w100:path, name=w98:string)
              n65 = Concatenate Strings("A_", w98) -> (w101:string)
              n66 = call "___save_2d_data_with_header.vi"("ヘッダー"="IF,Pout,p-p(31MHz)", "配列"=w102, "形式"="%.3f", "file_name"=w101, "パス"=w100) -> ()  [unwired: 6 in, 1 out]
            }
            frame #1 {
              n67 = local read "Totalband Power"() -> (w105:dbl)
              n68 = local read "Inband Power"() -> (w106:dbl)
              n69 = local read "Inband PP"() -> (w107:dbl)
              n70 = local read "max"() -> (w108:dbl)
              n71 = Format Into String(format string="SP_spurious,%.2f,%.2f,%.2f,%.2f ", w108, w107, w106, w105) -> (resulting string=w109:string)  [unwired: 2 in, 1 out]
              n72 = local write "出力文字列"(w109) -> ()
            }
          }
        }
      }
    }
  }
